vi "properties.get.vi"   [LabVIEW 2020, in "type.lvclass"]
uses:
  type.lvclass
  createdAt.get.vi
  datasourceConfigs.get.vi
  description.get.vi
  iconName.get.vi
  name.get.vi
  propertyConfigs.get.vi
  rid.get.vi
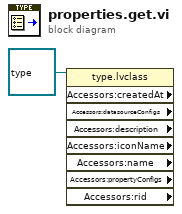
[diagram p0: block diagram]
diagram:
  n1 = property class="type.lvclass" props=["Accessors:createdAt", "Accessors:datasourceConfigs", "Accessors:description", "Accessors:iconName", "Accessors:name", "Accessors:propertyConfigs", "Accessors:rid"](reference=refnum<class "type.lvclass"> refnum ("type.lvclass")) -> ()  [unwired: 1 in, 9 out]
